vi "PCO_SetStorageMode.vi"(8 "error in (no error)":errorcluster, 10 "wStorageMode":enum16{"recorder", "fifo"}(ring), 11 "Handle":u64) -> (0 "error out":errorcluster, 3 "Handle Out":u64, 5 "return type":u32 format="%x")   [LabVIEW 2011]
uses:
  SC2_Cam64.dll
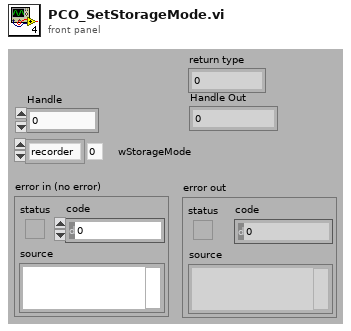
[diagram p1: front panel]
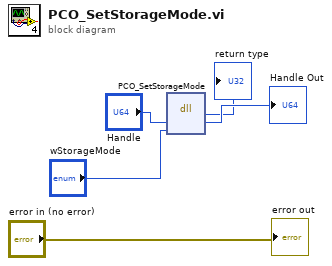
[diagram p0: block diagram]
diagram:
  n1 = dll-call lib="SC2_Cam*.*" fn="PCO_SetStorageMode"("Handle"="Handle", "wStorageMode"="wStorageMode") -> ("return type"=→"return type":u32, "Handle"=→"Handle Out":u64)  [unwired: 3 in, 3 out]
  "error out" <- "error in (no error)"
